vi "Temperature Warnings.vi"(8 "Error In":errorcluster, 9 "Min Temperature":dbl, 10 "Max Temperature":dbl, 11 "Current Temperature":dbl) -> (0 "Error Out":errorcluster, 2 "Warning Text":string="No Warning", 3 "Warning?":bool)   [LabVIEW 2015]
doc: "This VI is used to determine the string to output to the weather station based on the current temperature and limit settings.\n\nInputs: Current Temperature (DBL), Minimum Temperature (DBL), and Maximum Temperature (DBL).\nOutputs: Warning Text (string) and Warning? (Boolean)."
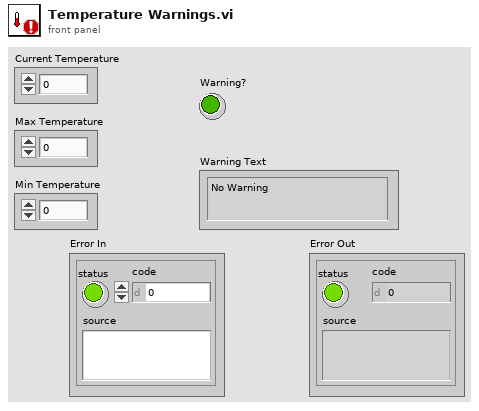
[diagram p1: front panel]
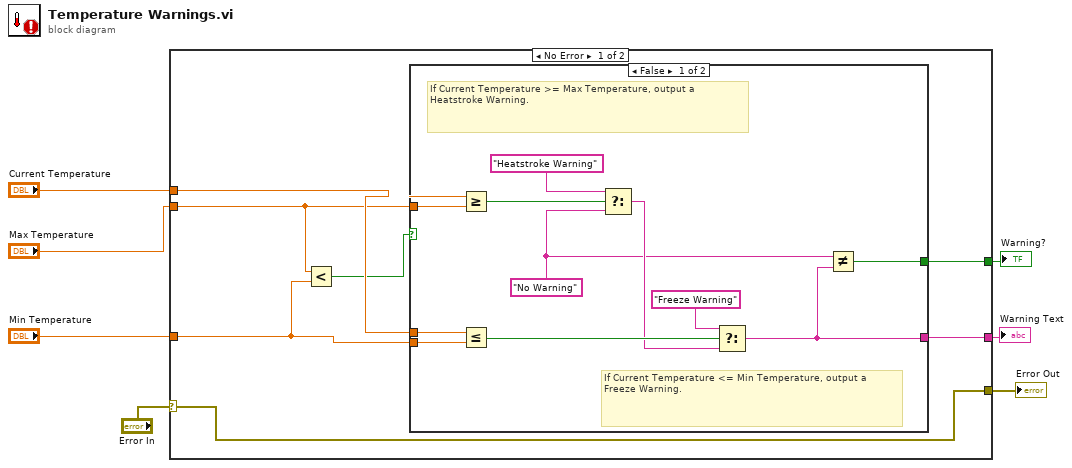
[diagram p0: block diagram]
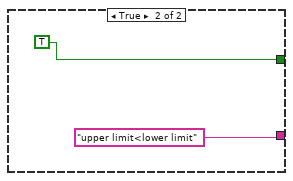
[diagram p2: hidden frame]
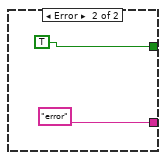
[diagram p3: hidden frame]
diagram:
  n1 = case shown="No Error" "Error In" {
    selector: "Error In" -> [w8 _]
    tunnel: "Min Temperature" -> [w13 _]
    tunnel: "Current Temperature" -> [w14 _]
    tunnel: "Max Temperature" -> [w12 _]
    tunnel: [w11 "error"] -> w4
    tunnel: [w10 TRUE] -> w3
    tunnel: [w8 _] -> w1
    frame No Error {
      n2 = Less?(x=w12, y=w13) -> (x < y?=w9:bool)
      n3 = case shown="False" w9 {
        tunnel: w14 -> [w19 _]
        tunnel: w13 -> [w18 _]
        tunnel: w12 -> [w17 _]
        tunnel: [w16 "upper limit<lower limit"] -> w11
        tunnel: [w15 TRUE] -> w10
        frame False {
          w20 = "No Warning" ("f")
          # "If Current Temperature >= Max Temperature, output a Heatstroke Warning."
          # "If Current Temperature <= Min Temperature, output a Freeze Warning."
          n4 = Greater Or Equal?(x=w19, y=w17) -> (x >= y?=w25:bool)
          n5 = Less Or Equal?(x=w19, y=w18) -> (x <= y?=w22:bool)
          n6 = Select(t="Heatstroke Warning", s=w25, f=w20) -> (s? t:f=w21:string)
          n7 = Select(t="Freeze Warning", s=w22, f=w21) -> (s? t:f=w16:string)
          n8 = Not Equal?(x=w20, y=w16) -> (x != y?=w15:bool)
        }
        frame True {
        }
      }
    }
    frame Error {
    }
  }
  "Error Out" <- w1
  "Warning?" <- w3
  "Warning Text" <- w4
